vi "1D Fit Rescale Fit Outputs.vi"(7 "Model Name":string, 8 "IRF Normalization Factor":dbl, 9 "Decay Normalization Factor":dbl, 10 "# Points":i32, 11 "Fit Output in":T1={"best nonlinear fit"=[], "best fit parameters"=[], "R^2"=0.0, "RMSE"=0.0, "error out"={"status"=FALSE, "code"=0, "source"=""}, "Fitting Method"=enum."Least Square", "number of function calls"=0, "number of iterations"=0, "covariance"=[], "Chi 2"=0.0, "DOF"=0, "Fit Convergence Criterion"=enum."Continue", "Fitting Algorithm"=enum."Levenberg-Marquardt", "Weighted Fit"=enum."Unweighted", "Gradient"=0.0, "|Delta Chi 2|"=0.0, "|Delta Chi 2|/Chi 2"=0.0, "Max |Delta a| /|a|"=0.0, "Lambda"=-1.0, "RSS"=0.0, "AIC"=0.0, "BIC"=0.0, "Max number of function calls"=0, "Max number of iterations"=0, "IRF"={"X Array"=[], "Y Array"=[]}, "IRF Normalization Factor"=0.0, "Decay Normalization Factor"=0.0, "Number of offset fits"=0, "Weighted Chi2"=-1.0, "Unweighted Chi2"=-1.0}) -> (3 "Fit Output out":T1={"best nonlinear fit"=[], "best fit parameters"=[], "R^2"=0.0, "RMSE"=0.0, "error out"={"status"=FALSE, "code"=0, "source"=""}, "Fitting Method"=enum."Least Square", "number of function calls"=0, "number of iterations"=0, "covariance"=[], "Chi 2"=0.0, "DOF"=0, "Fit Convergence Criterion"=enum."Continue", "Fitting Algorithm"=enum."Levenberg-Marquardt", "Weighted Fit"=enum."Unweighted", "Gradient"=0.0, "|Delta Chi 2|"=0.0, "|Delta Chi 2|/Chi 2"=0.0, "Max |Delta a| /|a|"=0.0, "Lambda"=-1.0, "RSS"=0.0, "AIC"=0.0, "BIC"=0.0, "Max number of function calls"=0, "Max number of iterations"=0, "IRF"={"X Array"=[], "Y Array"=[]}, "IRF Normalization Factor"=0.0, "Decay Normalization Factor"=0.0, "Number of offset fits"=0, "Weighted Chi2"=-1.0, "Unweighted Chi2"=-1.0})   [LabVIEW 2021, in "Fits.lvlib"]
uses:
  Fits.lvlib
  Non-linear Fit Output v4.ctl
  Nonlinear Fit Method.ctl
  <vilib>/Analysis/Matrix/Datatypes/RealMatrix.ctl
  Convergence Criteria.ctl
  Non-linear Fitting Algorithm.ctl
  IRF(X)PSED/Fit Weights Type v2.ctl
  Graphs/XY Graph/XY Graph Plot Data.ctl
  <vilib>/Analysis/Matrix/Numeric/Multiply/Multiply - RM,R.vi
  <vilib>/Analysis/Matrix/NI_Matrix.lvlib
  Graphs/XY Graph/XY Graph Add-Ons.lvlib
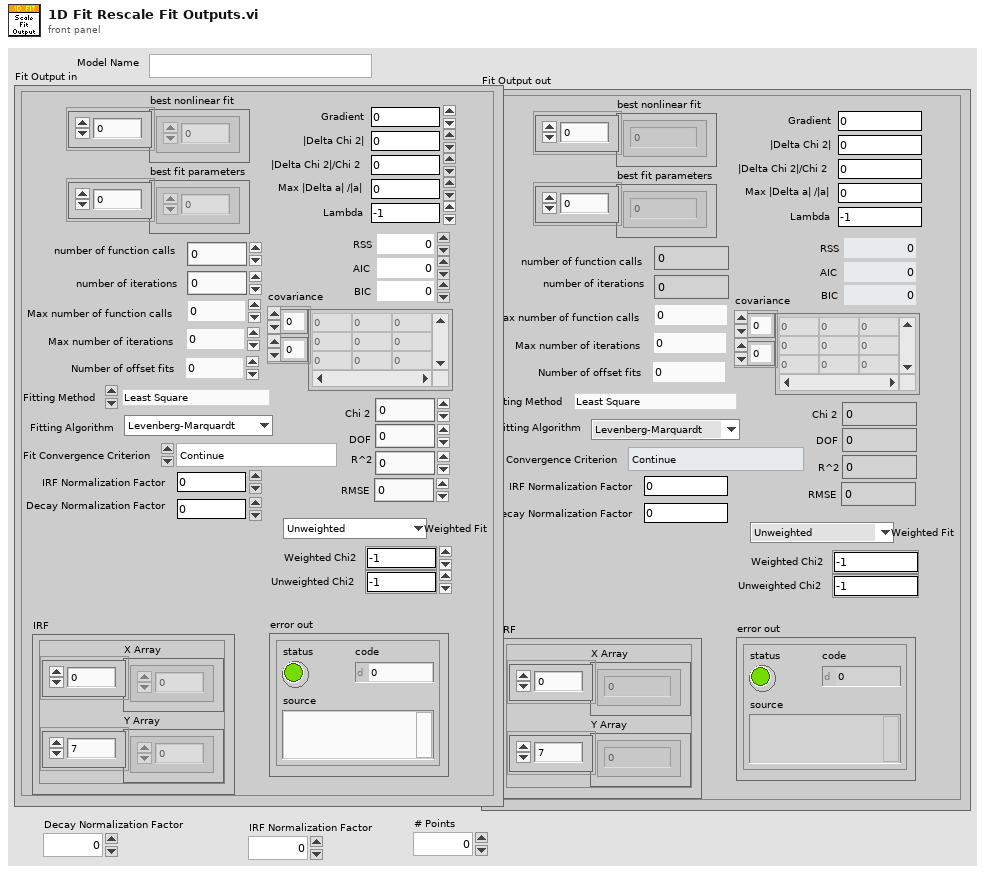
[diagram p1: front panel]
types:
  T1 = typedef "Fits.lvlib/Non-linear Fit Output v4.ctl" = cluster{"best nonlinear fit":dbl[], "best fit parameters":dbl[], "R^2":dbl, "RMSE":dbl, "error out":errorcluster, "Fitting Method":T2, "number of function calls":i32, "number of iterations":i32, "covariance":T3, "Chi 2":dbl, "DOF":i32, "Fit Convergence Criterion":T4, "Fitting Algorithm":T5, "Weighted Fit":T6, "Gradient":dbl, "|Delta Chi 2|":dbl, "|Delta Chi 2|/Chi 2":dbl, "Max |Delta a| /|a|":dbl, "Lambda":dbl, "RSS":dbl, "AIC":dbl, "BIC":dbl, "Max number of function calls":i32, "Max number of iterations":i32, "IRF":T7, "IRF Normalization Factor":dbl, "Decay Normalization Factor":dbl, "Number of offset fits":i32, "Weighted Chi2":dbl, "Unweighted Chi2":dbl}
  T2 = typedef "Fits.lvlib/Nonlinear Fit Method.ctl" = enum16{"Least Square", "Least Absolute Residual", "Bisquare", "MLE"}
  T3 = typedef "NI_Matrix.lvlib/RealMatrix.ctl" = dbl[][]
  T4 = typedef "Fits.lvlib/Convergence Criteria.ctl" = enum16{"Continue", "Tolerances Exceeded", "Max Time Exceeded", "Max Iterations Exceeded", "Max Function Evaluations Exceeded", "Scale Range Exceeded"}
  T5 = typedef "Fits.lvlib/Non-linear Fitting Algorithm.ctl" = enum16{"Levenberg-Marquardt", "Trust-Region Dogleg"}
  T6 = typedef "Fits.lvlib/Fit Weights Type v2.ctl" = enum16{"Unweighted", "1/Variance (Neyman)", "1/Variance (Pearson)", "Best of All"}
  T7 = typedef "XY Graph Add-Ons.lvlib/XY Graph Plot Data.ctl" = cluster{"X Array":dbl[], "Y Array":dbl[]}
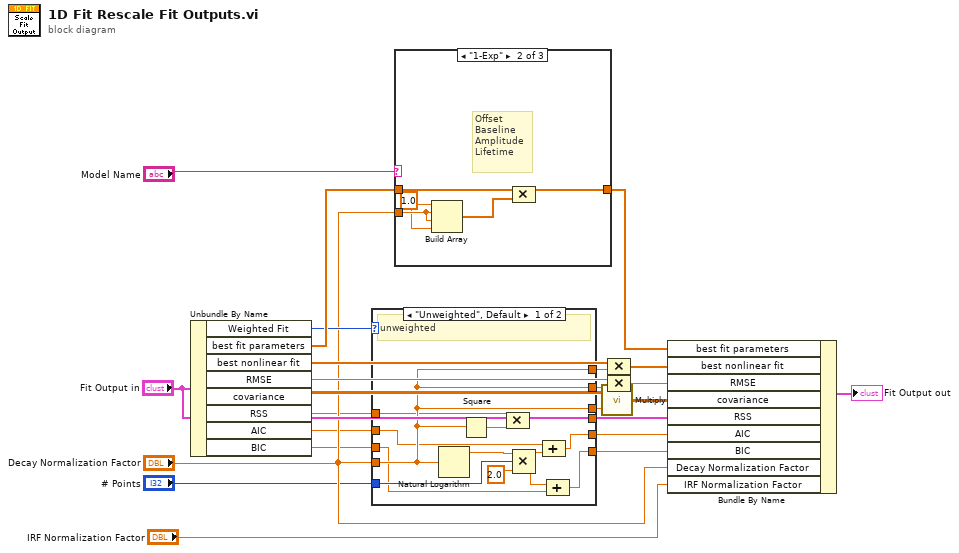
[diagram p0: block diagram]
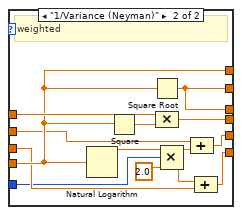
[diagram p2: hidden frame]
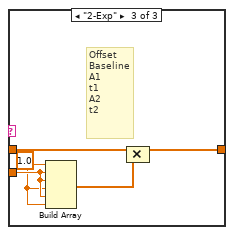
[diagram p4: hidden frame]
diagram:
  n1 = Unbundle By Name("Fit Output in") -> ("Weighted Fit"=w10:T6, "best fit parameters"=w12:dbl[], "best nonlinear fit"=w22:dbl[], "RMSE"=w20:dbl, "covariance"=w18:T3, "RSS"=w7:dbl, "AIC"=w6:dbl, "BIC"=w5:dbl)
  n2 = case shown="\"Unweighted\", Default" w10 {
    tunnel: "Decay Normalization Factor" -> [w32 w43]
    tunnel: [w32 w43] -> w17
    tunnel: [w32 w49] -> w16
    tunnel: [w32 w49] -> w15
    tunnel: w7 -> [w30 w44]
    tunnel: w6 -> [w28 w42]
    tunnel: w5 -> [w25 w41]
    tunnel: "# Points" -> [w31 w40]
    tunnel: [w29 w39] -> w3
    tunnel: [w27 w38] -> w2
    tunnel: [w26 w37] -> w1
    frame "Unweighted", Default {
      # "unweighted"
      n3 = Natural Logarithm(1:w32) -> (0:w35:dbl)
      n4 = Square(x=w32) -> (x^2=w36:dbl)
      n5 = Compound Arithmetic op=MULTIPLY(w30, w36) -> (w29:dbl)
      n6 = Compound Arithmetic op=MULTIPLY(w35, w31, 2.0 ("value")) -> (w33:dbl)
      n7 = Compound Arithmetic op=ADD(w28, w33) -> (w27:dbl)
      n8 = Compound Arithmetic op=ADD(w33, w25) -> (w26:dbl)
    }
    frame "1/Variance (Neyman)" {
      # "weighted"
      n9 = Natural Logarithm(1:w43) -> (0:w47:dbl)
      n10 = Square(x=w43) -> (x^2=w48:dbl)
      n11 = Square Root(x=w43) -> (sqrt(x)=w49:dbl)
      n12 = Compound Arithmetic op=MULTIPLY(w44, w48) -> (w39:dbl)
      n13 = Compound Arithmetic op=MULTIPLY(w47, w40, 2.0 ("value")) -> (w45:dbl)
      n14 = Compound Arithmetic op=ADD(w42, w45) -> (w38:dbl)
      n15 = Compound Arithmetic op=ADD(w45, w41) -> (w37:dbl)
    }
  }
  n16 = case shown="\"1-Exp\"" "Model Name" {
    tunnel: w12 -> [w50 w53 w60]
    tunnel: [w50 w51 w58] -> w11
    tunnel: "Decay Normalization Factor" -> [_ w55 w57]
    frame "", Default {
      # "undefined parameter scaling"
    }
    frame "1-Exp" {
      w54 = 1.0 ("element")
      # "Offset\nBaseline\nAmplitude\nLifetime"
      n17 = Build Array(w54, w55, w55, w54) -> (w52:dbl[])
      n18 = Compound Arithmetic op=MULTIPLY(w53, w52) -> (w51:dbl[])
    }
    frame "2-Exp" {
      w56 = 1.0 ("element")
      # "Offset\nBaseline\nA1\nt1\nA2\nt2"
      n19 = Build Array(w56, w57, w57, w56, w57, w56) -> (w59:dbl[])
      n20 = Compound Arithmetic op=MULTIPLY(w60, w59) -> (w58:dbl[])
    }
  }
  n21 = call-poly <vilib>:"Multiply.vi"("Real Scalar c"=w15, "Real Matrix A"=w18) -> ("A * c"=w14:T3)
  n22 = Compound Arithmetic op=MULTIPLY(w22, w17) -> (w21:dbl[])
  n23 = Compound Arithmetic op=MULTIPLY(w20, w16) -> (w19:dbl)
  n24 = Bundle By Name(cluster="Fit Output in", "best fit parameters"=w11, "best nonlinear fit"=w21, "RMSE"=w19, "covariance"=w14, "RSS"=w3, "AIC"=w2, "BIC"=w1, "Decay Normalization Factor"="Decay Normalization Factor", "IRF Normalization Factor"="IRF Normalization Factor") -> (→"Fit Output out":T1)
